vi "Delete File and Folder.vi"(8 "error in (no error)":errorcluster, 11 "Path":path) -> (0 "error out":errorcluster)   [LabVIEW 2019, in "ProjectItem.lvclass"]
uses:
  ProjectItem.lvclass
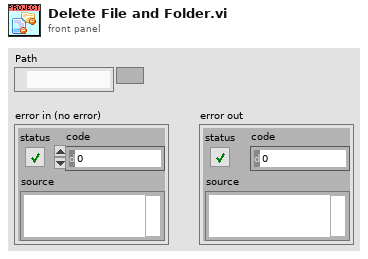
[diagram p1: front panel]
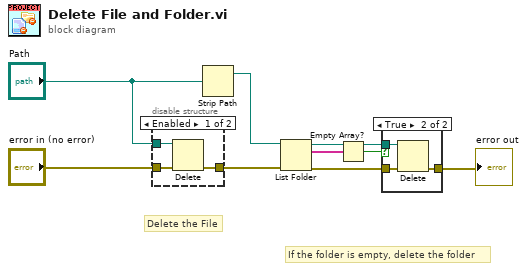
[diagram p0: block diagram]
diagram:
  # "If the folder is empty, delete the folder"
  # "Delete the File"
  n1 = disable-structure shown="Enabled" {
    disable-tunnel: "Path" -> [w12 _]
    disable-tunnel: "error in (no error)" -> [w11 w13]
    disable-tunnel: [w10 w13] -> w8
    frame Enabled {
      n2 = Delete(path (use dialog)=w12, error in=w11) -> (error out=w10:errorcluster)  [unwired: 3 in, 2 out]
    }
    frame Disabled {
    }
  }
  n3 = Strip Path(path="Path") -> (stripped path=w7:path)  [unwired: 1 out]
  n4 = List Folder(path=w7, error in=w8) -> (path out=w3:path, filenames=w2:string[], error out=w4:errorcluster)  [unwired: 2 in, 1 out]
  n5 = Empty Array?(array=w2) -> (empty?=w5:bool)
  n6 = case shown="True" w5 {
    tunnel: w3 -> [_ w17]
    tunnel: w4 -> [w14 w16]
    tunnel: [w14 w15] -> w9
    frame False {
    }
    frame True {
      n7 = Delete(path (use dialog)=w17, error in=w16) -> (error out=w15:errorcluster)  [unwired: 3 in, 2 out]
    }
  }
  "error out" <- w9
